vi "MHTML Binary Section.vi"(4 "boundary":string, 5 "error in (no error)":errorcluster, 8 "attachment":path) -> (0 "error out":errorcluster, 3 "MHTML Attachment":string)   [LabVIEW 2011]
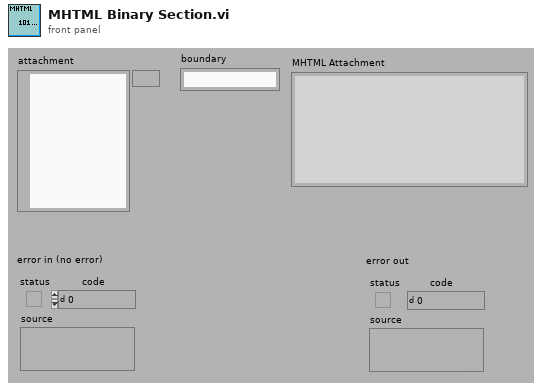
[diagram p1: front panel]
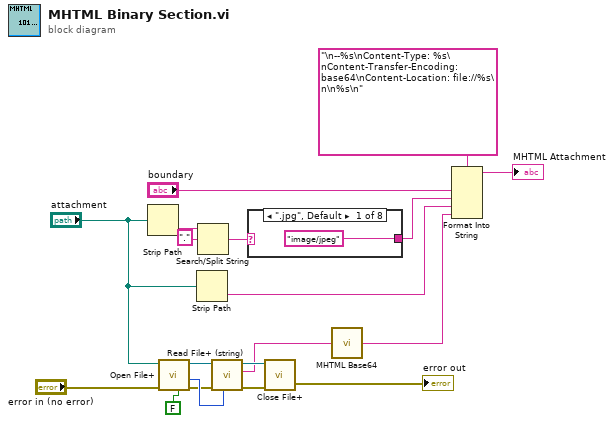
[diagram p0: block diagram]
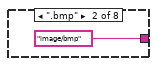
[diagram p2: hidden frame]
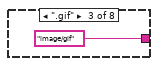
[diagram p3: hidden frame]
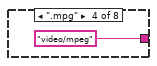
[diagram p4: hidden frame]
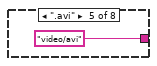
[diagram p5: hidden frame]
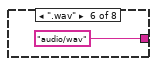
[diagram p6: hidden frame]
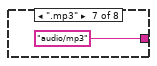
[diagram p7: hidden frame]
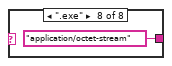
[diagram p8: hidden frame]
diagram:
  n1 = Strip Path(path="attachment") -> (name=w18:string)  [unwired: 1 out]
  n2 = call <vilib>:"Open File+.vi"("advisory dialog? (display:T)"=FALSE, "error in (not an error)"="error in (no error)", "file path (\" \")"="attachment") -> ("error out"=w9:errorcluster, "file size (bytes)"=w10:i32, "refnum"=w5:refnum<file>)  [unwired: 4 in, 2 out]
  n3 = Strip Path(path="attachment") -> (name=w1:string)  [unwired: 1 out]
  n4 = Search/Split String(string=w18, search string/char (-)=".") -> (match + rest of string=w16:string)  [unwired: 3 out]
  n5 = call <vilib>:"Read File+ (string).vi"("count"=w10, "error in (no error)"=w9, "refnum"=w5) -> ("error out"=w8:errorcluster, "string"=w3:string, "dup refnum"=w4:refnum<file>)  [unwired: 2 in, 4 out]
  n6 = case shown="\".jpg\", Default" w16 {
    tunnel: ["image/jpeg" "image/bmp" "image/gif" "video/mpeg" "video/avi" "audio/wav" "audio/mp3" "application/octet-stream"] -> w15
    frame ".jpg", Default {
    }
    frame ".bmp" {
    }
    frame ".gif" {
    }
    frame ".mpg" {
    }
    frame ".avi" {
    }
    frame ".wav" {
    }
    frame ".mp3" {
    }
    frame ".exe" {
    }
  }
  n7 = call <vilib>:"Close File+.vi"("error in (no error)"=w8, "refnum"=w4) -> ("error out"=→"error out":errorcluster)  [unwired: 5 out]
  n8 = call "MHTML Base64.vi"("Binary String"=w3) -> ("String (Base64)"=w14:string)  [unwired: 14 out]
  n9 = Format Into String(format string="\n--%s\nContent-Type: %s\nContent-Transfer-Encoding: base64\nContent-Location: file://%s\n\n%s\n", "boundary", w15, w1, w14) -> (resulting string=→"MHTML Attachment":string)  [unwired: 2 in, 1 out]
